vi "SaveDataSet_SpeedProfile.vi"(6 "AssetNodeMap":variant, 7 "do not write to database":bool, 8 "error in (no error)":errorcluster, 9 "speed profile":sgl[](array[numeric]), 10 "DataSetRegistry":T1, 11 "event in":T3) -> (0 "error out":errorcluster, 3 "event out":T3)   [LabVIEW 2017, in "CmsDataEventCreator.lvlib"]
uses:
  <vilib>/addons/InsightCM/Devices/Shared/Cms/CmsDataEventCreator/CmsDataEventCreator.lvlib
  <vilib>/addons/InsightCM/Devices/Shared/Common/DataEvent/controls/Event.ctl
  <vilib>/addons/InsightCM/MessageBus/Base/controls/DataEvent.ctl
  <vilib>/addons/InsightCM/MessageBus/Base/controls/KeyValuePair.ctl
  <vilib>/addons/InsightCM/Devices/Shared/Common/DataEvent/controls/DataSet.ctl
  <vilib>/addons/InsightCM/MessageBus/Base/controls/DataSetMetadata.ctl
  <vilib>/addons/InsightCM/MessageBus/Base/controls/TrendPoint.ctl
  <vilib>/addons/InsightCM/MessageBus/Base/controls/TrendAlarmUpdate.ctl
  <vilib>/addons/InsightCM/MessageBus/Base/controls/TrendAlarmTransition.ctl
  <vilib>/addons/InsightCM/Devices/Shared/Cms/CmsDataEventCreator/controls/DataSetRegistry.ctl
  <vilib>/addons/InsightCM/Devices/Shared/Common/DataEvent/controls/DataSetType.ctl
  <vilib>/addons/InsightCM/Devices/Shared/Common/DataEventCreator/DataEventCreator.lvlib
  <vilib>/addons/InsightCM/Devices/Shared/Common/DataEvent/DataEvent.lvlib
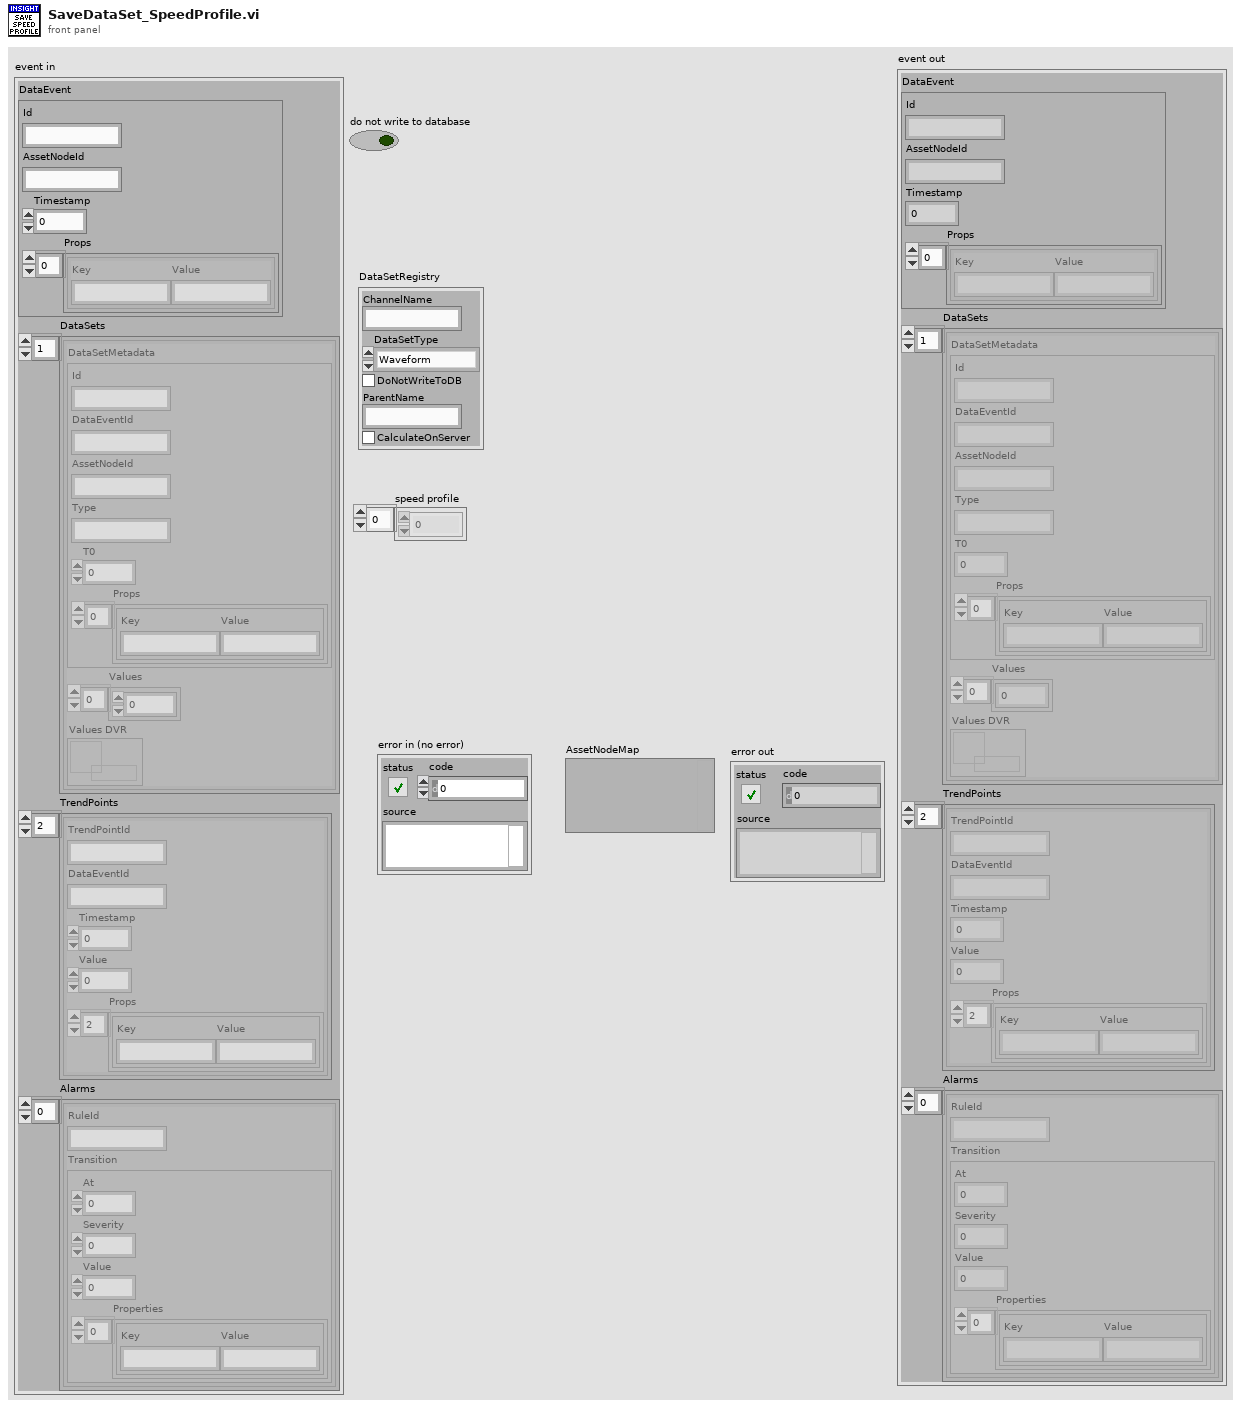
[diagram p1: front panel]
types:
  T1 = typedef "CmsDataEventCreator.lvlib/DataSetRegistry.ctl" = cluster{"ChannelName":string, "DataSetType":T2, "DoNotWriteToDB":bool, "ParentName":string, "CalculateOnServer":bool}
  T2 = typedef "DataEvent.lvlib/DataSetType.ctl" = enum16{"Waveform", "SpeedProfile", "ThermalImage", "EmsaSweep"}
  T3 = typedef "DataEvent.lvlib/Event.ctl" = cluster{"DataEvent":T4, "DataSets":T6[], "TrendPoints":T8[], "Alarms":T9[]}
  T4 = typedef "DataEvent.ctl" = cluster{"Id":string, "AssetNodeId":string, "Timestamp":i64, "Props":T5[]}
  T5 = typedef "KeyValuePair.ctl" = cluster{"Key":string, "Value":string}
  T6 = typedef "DataEvent.lvlib/DataSet.ctl" = cluster{"DataSetMetadata":T7, "Values":sgl[], "Values DVR":refnum<data-value>}
  T7 = typedef "DataSetMetadata.ctl" = cluster{"Id":string, "DataEventId":string, "AssetNodeId":string, "Type":string, "T0":i64, "Props":T5[]}
  T8 = typedef "TrendPoint.ctl" = cluster{"TrendPointId":string, "DataEventId":string, "Timestamp":i64, "Value":dbl, "Props":T5[]}
  T9 = typedef "TrendAlarmUpdate.ctl" = cluster{"RuleId":string, "Transition":T10}
  T10 = typedef "TrendAlarmTransition.ctl" = cluster{"At":i64, "Severity":i32, "Value":dbl, "Properties":T5[]}
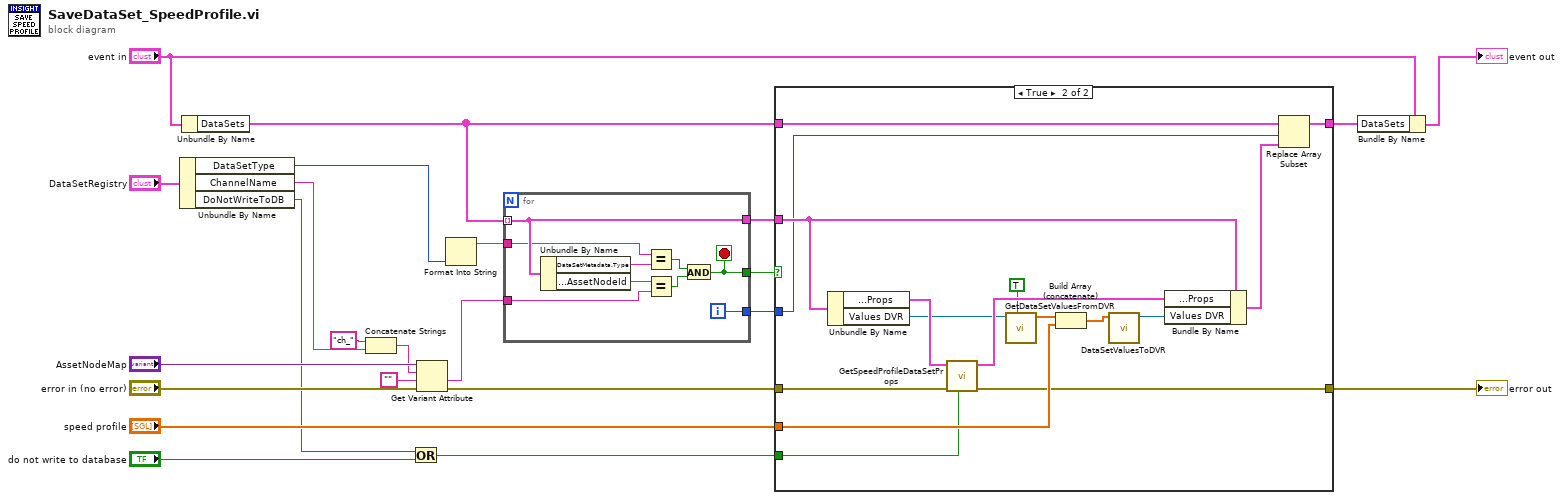
[diagram p0: block diagram]
diagram:
  n1 = Unbundle By Name("DataSetRegistry") -> ("DataSetType"=w9:T2, "ChannelName"=w2:string, "DoNotWriteToDB"=w6:bool)
  n2 = Unbundle By Name("event in") -> ("DataSets"=w11:T6[])
  n3 = Concatenate Strings("ch_" ("string"), w2) -> (w1:string)
  n4 = Or(x=w6, y="do not write to database") -> (x .or. y?=w4:bool)
  n5 = Get Variant Attribute(Variant="AssetNodeMap", name=w1, default value (empty Variant)="", error in="error in (no error)") -> (value=w8:string, error out=w15:errorcluster)  [unwired: 2 out]
  n6 = Format Into String(w9) -> (resulting string=w7:string)  [unwired: 3 in, 1 out]
  n7 = for {
    tunnel: w11 -> [w30] mode=indexing
    tunnel: w8 -> [w31]
    tunnel: [w26] -> w12
    tunnel: [w30] -> w10
    tunnel: [w29] -> w13
    tunnel: w7 -> [w24]
    i -> [w29]
    stop <- w26 stop-if-true
    n8 = Unbundle By Name(w30) -> ("DataSetMetadata.Type"=w25:string, "DataSetMetadata.AssetNodeId"=w32:string)
    n9 = Equal?(x=w24, y=w25) -> (x = y?=w28:bool)
    n10 = Equal?(x=w32, y=w31) -> (x = y?=w27:bool)
    n11 = And(x=w28, y=w27) -> (x .and. y?=w26:bool)
  }
  n12 = case shown="True" w12 {
    tunnel: w15 -> [w33 w44]
    tunnel: "speed profile" -> [_ w50]
    tunnel: w11 -> [w34 w48]
    tunnel: [w34 w47] -> w19
    tunnel: w10 -> [_ w49]
    tunnel: w13 -> [_ w46]
    tunnel: [w33 w43] -> w14
    tunnel: w4 -> [_ w42]
    frame False {
    }
    frame True {
      n13 = Unbundle By Name(w49) -> ("DataSetMetadata.Props"=w41:T5[], "Values DVR"=w39:refnum<data-value>)
      n14 = call <vilib>:"GetSpeedProfileDataSetProps.vi"("do not write to database"=w42, "error in (no error)"=w44, "dataset props in"=w41) -> ("error out"=w43:errorcluster, "dataset props out"=w40:T5[])  [unwired: 7 in]
      n15 = call <vilib>:"GetDataSetValuesFromDVR.vi"("delete dvr"=TRUE, "values dvr"=w39) -> ("values"=w37:sgl[])  [unwired: 8 in, 1 out]
      n16 = Build Array (concatenate)(w37, w50) -> (w36:sgl[])
      n17 = call <vilib>:"DataSetValuesToDVR.vi"("dataset values"=w36) -> ("new dataset values dvr"=w35:refnum<data-value>)  [unwired: 9 in, 1 out]
      n18 = Bundle By Name(cluster=w49, "DataSetMetadata.Props"=w40, "Values DVR"=w35) -> (w45:T6)
      n19 = Replace Array Subset(array=w48, new element=w45, index=w46) -> (w47:T6[])
    }
  }
  "error out" <- w14
  n20 = Bundle By Name(cluster="event in", "DataSets"=w19) -> (→"event out":T3)
